vi "RT Main51.vi"() -> ()   [LabVIEW 2019]
uses:
  <vilib>/FPGAPlugInAG/ELVIS III/niLvFpga_Open_ELVIS III.vi
  <vilib>/rvi/interface/common/dynamic/niFpgaDynamicAddResources.vi
  <vilib>/myRIO/Common/Instrument Driver Framework/Utilities/vis/FPGA Ref Manager.vi
  <vilib>/Utility/error.llb/Error Cluster From Error Code.vi
  <vilib>/myRIO/Common/Instrument Driver Framework/Utilities/vis/Ref Counter.vi
  <vilib>/rvi/errors/niLvFpgaAdjustHostInterfaceError.vi
  <vilib>/FPGAPlugInAG/Dynamic/niLvFpga_Close_Dynamic.vi
  <vilib>/rvi/interface/nirviOpenFPGA/nirviOpenFPGA.xnode
  FPGA Bitfiles/measurementpwmfr_FPGATarget_PWM5_dVHC8fwqfPA.lvbitx
  PWM5.vi
  <vilib>/rvi/interface/nirviReadWriteControl/nirviReadWriteControl.xnode
  <vilib>/rvi/interface/nirviCloseFPGA/nirviCloseFPGA.xnode
  <vilib>/myRIO/Instrument Drivers/Utilities/Utilities.lvlib
  NiFpgaLv.dll
  <vilib>/rvi/interface/Simulation/niFpgaSimulationCallBeginRW.vi
panel:
  out "x/y":dbl format="%#_10g"
  out "error out":errorcluster
  in  "Stop":bool
  out "波形图表":dbl(graph)
  out "数值":dbl
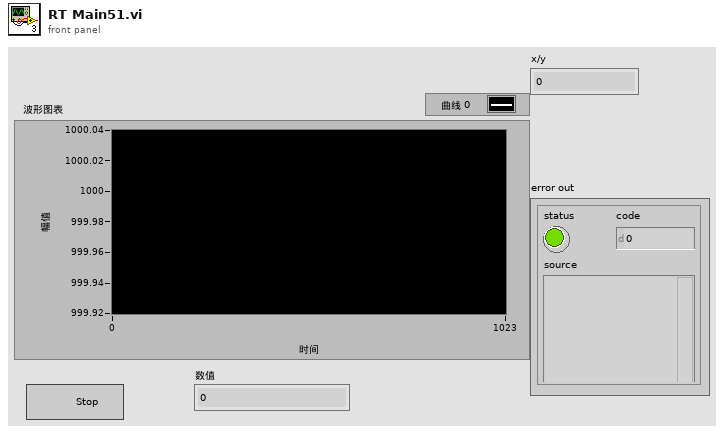
[diagram p1: front panel]
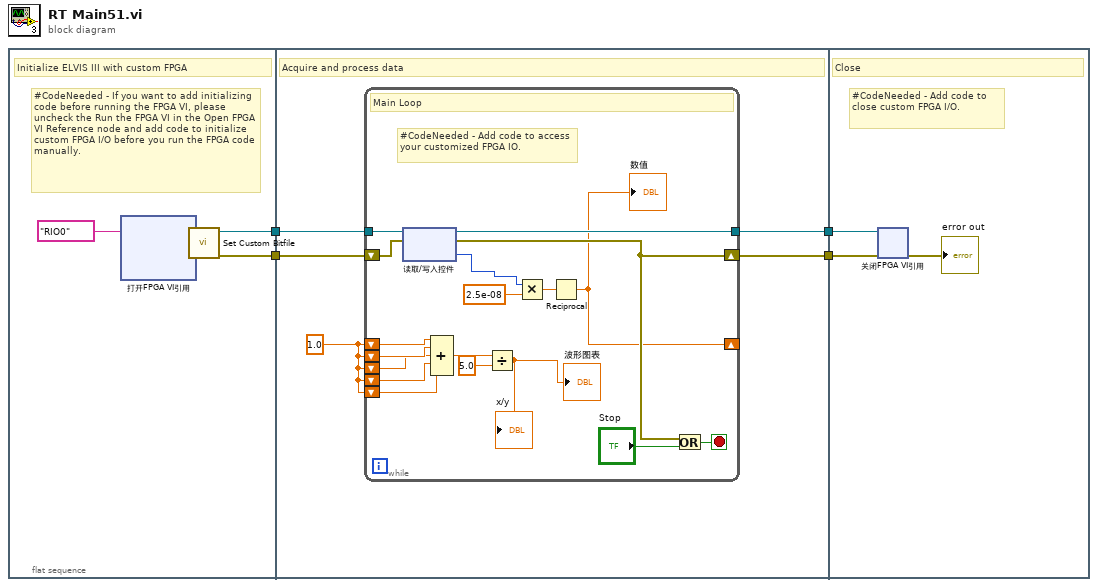
[diagram p0: block diagram]
diagram:
  n1 = flat-sequence {
    tunnel: [w6] -> w4
    tunnel: [w7] -> w3
    tunnel: w4 -> [w14]
    tunnel: w3 -> [w13]
    tunnel: [w12] -> w2
    tunnel: [w11] -> w1
    tunnel: w2 -> [w35]
    tunnel: w1 -> [w34]
    frame #0 {
      # "#CodeNeeded - If you want to add initializing code before running the FPGA VI, please uncheck the Run the FPGA VI in the Open FPGA VI Reference node and add code to initialize custom FPGA I/O before you run the FPGA code manually."
      # "Initialize ELVIS III with custom FPGA"
      n2 = xnode "打开FPGA VI引用"("资源名称"=tag "RIO0" ("resource name")) -> ("FPGA VI引用输出"=w8:refnum<k20>, "错误输出"=w9:errorcluster)  [unwired: 1 in]
      n3 = call <vilib>:"Set Custom Bitfile.vi"("error in (no error)"=w9, "Custom FPGA Reference In"=w8) -> ("error out"=w6:errorcluster, "Custom FPGA Reference Out"=w7:refnum<k20>)  [unwired: 8 in]
    }
    frame #1 {
      w10 = 1.0
      # "Acquire and process data"
      n4 = while {
        tunnel: w13 -> [w30]
        tunnel: [w29] -> w12
        shift-right: [w27] -> w11
        shift-left: w14 -> [w28]
        shift-right: [w23] -> _
        shift-left: w10 -> [w22]
        shift-left: w10 -> [w21]
        shift-left: w10 -> [w20]
        shift-left: w10 -> [w19]
        shift-left: w10 -> [w18]
        stop <- w31 stop-if-true
        # "#CodeNeeded - Add code to access your customized FPGA IO."
        # "Main Loop"
        n5 = xnode "读取/写入控件"("FPGA VI引用输入"=w30, "错误输入"=w28) -> ("FPGA VI引用输出"=w29:refnum<k20>, "错误输出"=w27:errorcluster, "x-1"=w24:u32)
        n6 = Compound Arithmetic op=ADD ("复合运算")(w22, w21, w20, w19, w18) -> (w17:dbl)
        n7 = Divide(x=w17, y=5.0) -> (x/y=→"波形图表" →"x/y":dbl)
        n8 = Multiply(x=w24, y=2.5e-08) -> (x*y=w26:dbl)
        n9 = Reciprocal(x=w26) -> (1/x=w23:dbl)
        "数值" <- w23
        n10 = Or(x=w27, y="Stop") -> (x .or. y?=w31:bool)
      }
    }
    frame #2 {
      # "#CodeNeeded - Add code to close custom FPGA I/O."
      # "Close"
      n11 = xnode "关闭FPGA VI引用"("FPGA VI引用输入"=w35, "错误输入"=w34) -> ("错误输出"=→"error out":errorcluster)
    }
  }
